vi "sosfilter.vi"() -> ()   [LabVIEW 2015]
uses:
  <vilib>/Platform/TimedLoop/XDataNode/timing_clust.ctl
  <vilib>/Platform/TimedLoop/XDataNode/nitl_modes.ctl
  <vilib>/Platform/TimedLoop/XDataNode/wakeup.ctl
  <vilib>/rvi/Emulation/niFpgaGetClockAttributes.vi
  <vilib>/rvi/Emulation/niFpgaSctlEmulationGetInTimedLoop.vi
  <vilib>/rvi/Emulation/niFpgaEmulationReportErrorSimple.vi
  <vilib>/rvi/eio/common/nirviEmuTemplateMethod_errors.vi
  <vilib>/rvi/Emulation/niFpgaEmulationIsFPGAContextNoSignature.vi
  <vilib>/rvi/errors/niFpgaSetErrorForExecOnDevCompSimple.vi
  <vilib>/rvi/eio/common/nirviEmuReportErrorAndStop.vi
  <vilib>/rvi/DataTransferAndStorage/Container/Common/niFpgaContainerGetUniqueNameForEmu.vi
  <vilib>/rvi/FIFO/Fifo_Resource/nirvififoEmulationSetSize.vi
  <vilib>/rvi/FIFO/Fifo_Resource/nirviFifoEmulationQueueMgr.vi
  <instcachedir>/0/nirviFifoEmulationQueueMgr_E5CAEC123FF24DC58D834DCA3CDAA9B5.lvgen/nirviFifoEmulationQueueMgr_E5CAEC123FF24DC58D834DCA3CDAA9B5_017.vi
  <vilib>/rvi/FIFO/Fifo_Resource/nirvififoEmulationDetermineInputValidOut.vi
  <vilib>/rvi/FIFO/Fifo_Resource/nirvififoEmulationCreateLock.vi
  <vilib>/rvi/Emulation/niFpgaProcessEmulError.vi
  <vilib>/rvi/FIFO/Fifo_Resource/nirvififoEmulationObtainLock.vi
  <vilib>/rvi/FIFO/Fifo_Resource/nirvififoEmulationReleaseLock.vi
  <vilib>/rvi/occurrence/nirviWaitOnOccurrenceBase.vi
  <vilib>/rvi/errors/nirviReportUnexpectedCaseInternalError.vi
  <vilib>/rvi/errors/nirviReportUnexpectedCaseInternalError (U32).vi
  <vilib>/rvi/Emulation/niFpgaCriticalErrorInLSC.vi
  <instcachedir>/0/nirviFifoEmulationQueueMgr_E5CAEC123FF24DC58D834DCA3CDAA9B5.lvgen/nirviFifoEmulationQueueMgr_E5CAEC123FF24DC58D834DCA3CDAA9B5_008.vi
  <vilib>/Utility/error.llb/Clear Errors.vi
  <vilib>/eio/EIONode/EIONode.xnode
  <vilib>/rvi/DataTransferAndStorage/Container/XNode/niFpgaContainer.xnode
  <vilib>/rvi/FIFO/Fifo_Resource/nirvififoEmulationWrite.vi
  <vilib>/rvi/FIFO/Fifo_Resource/nirvififoEmulationRead.vi
  <vilib>/Platform/TimedLoop/XDataNode/XDataNode.xnode
  <vilib>/rvi/FXPMathLib/FxpMul/XNode/nifxpmath_Multiplier.xnode
  <vilib>/rvi/FXPMathLib/FxpAdd/XNode/nifxpmath_Add.xnode
  <vilib>/Platform/TimedLoop/XDataNode/XDNodeRunTimeDep.lvlib
  <vilib>/rvi/FXPMathLib/sim/FxpSim.dll
panel:
  in  "a2":fxp<+/-,24,5>
  in  "b2":fxp<+/-,24,5>
  in  "b1":fxp<+/-,24,5>
  in  "a1":fxp<+/-,24,5>
  in  "b0":fxp<+/-,24,5>
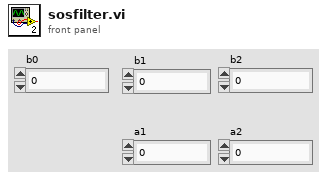
[diagram p1: front panel]
types:
  T1 = typedef "XDNodeRunTimeDep.lvlib/timing_clust.ctl" = cluster{"Expected End [f-1]":u64, "Actual End [f-1]":u64, "Finished Late? [f-1]":bool, "Expected End [i-1]":u64, "Actual End [i-1]":u64, "Finished Late? [i-1]":bool, "Expected Start [i]":u64, "Actual Start [i]":u64, "Expected Start [f]":u64, "Actual Start [f]":u64, "Source Name":string, "Structure Name":string, "Period":i64, "Deadline":i64, "Offset":i64, "Start":i64, "Priority":i32, "Timeout":i32, "Mode":T2, "Wakeup Reason":T3, "Error":errorcluster, "Source Type":string, "Secondary Source Type":string, "Global End Time":u64, "Global Start Time":u64, "Frame Duration":u64, "Iteration Duration":u64, "Assigned CPU":i32, "I/O Scan Engine Mode":u32}
  T2 = typedef "XDNodeRunTimeDep.lvlib/nitl_modes.ctl" = enum32{"No Change", "Process missed periods, maintain original phase", "Discard missed periods, maintain original phase", "Process missed periods, ignore original phase", "Discard missed periods, ignore original phase"}
  T3 = typedef "XDNodeRunTimeDep.lvlib/wakeup.ctl" = enum32{"Normal", "Aborted", "Asynchronous wakeup", "Timing source error", "Timed loop error", "Timeout"}
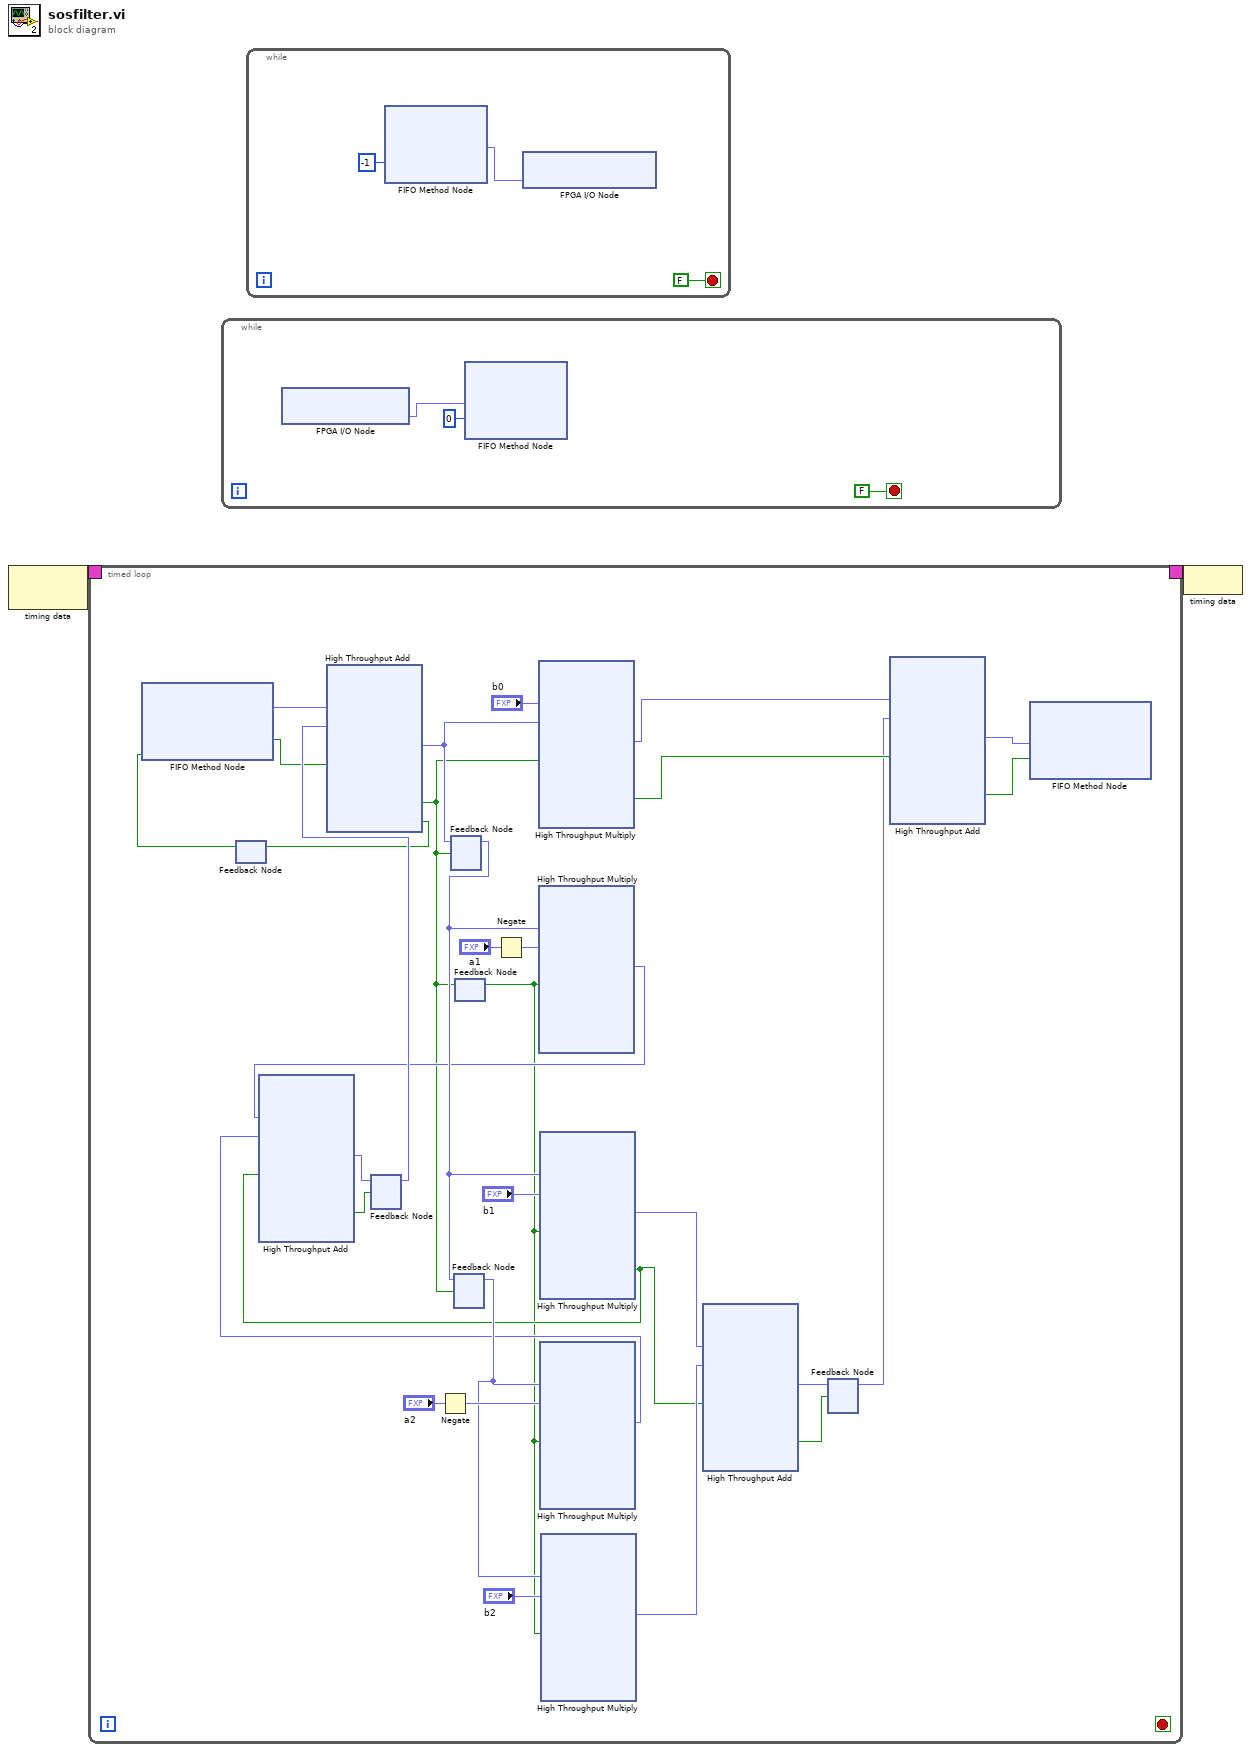
[diagram p0: block diagram]
diagram:
  n1 = node-c288() -> (w2:T1)  [unwired: 1 in]
  n2 = timed-loop {
    timing: w2 -> [_]
    timing-out: [_] -> w1
    stop <- _ stop-if-true
    n3 = feedback #1() -> (w7:bool)  [unwired: 1 in]
    n4 = xnode ("FIFO Method Node")("Ready for Output"=w7) -> ("Element"=w24:fxp<+/-,18,5>, "Output Valid"=w9:bool)  [unwired: 1 in, 1 out]
    n5 = feedback #2() -> (w19:fxp<+/-,36,16>)  [unwired: 1 in]
    n6 = xnode ("High Throughput Add")("x"=w24, "y"=w19, "input valid"=w9) -> ("x+y"=w23:fxp<+/-,36,16>, "output valid"=w13:bool, "ready for input"=w8:bool)  [unwired: 1 in]
    n7 = feedback-in #1(w8) -> ()
    n8 = Negate(x="a2") -> (-x=w27:fxp<+/-,25,6>)
    n9 = feedback-in #3(w23, w13) -> ()
    n10 = feedback #3() -> (w32:fxp<+/-,36,16>)  [unwired: 1 in]
    n11 = feedback #4() -> (w25:fxp<+/-,36,16>)  [unwired: 1 in]
    n12 = feedback-in #4(w32, w13) -> ()
    n13 = feedback-in #5(w13) -> ()
    n14 = feedback #5() -> (w12:bool)  [unwired: 1 in]
    n15 = Negate(x="a1") -> (-x=w30:fxp<+/-,25,6>)
    n16 = xnode ("High Throughput Multiply")("x"="b0", "y"=w23, "input valid"=w13) -> ("x*y"=w6:fxp<+/-,36,16>, "output valid"=w5:bool)  [unwired: 1 in, 1 out]
    n17 = xnode ("High Throughput Multiply")("x"=w32, "y"=w30, "input valid"=w12) -> ("x*y"=w18:fxp<+/-,36,16>)  [unwired: 1 in, 2 out]
    n18 = xnode ("High Throughput Multiply")("x"=w32, "y"="b1", "input valid"=w12) -> ("x*y"=w17:fxp<+/-,36,16>, "output valid"=w15:bool)  [unwired: 1 in, 1 out]
    n19 = xnode ("High Throughput Multiply")("x"=w25, "y"=w27, "input valid"=w12) -> ("x*y"=w22:fxp<+/-,36,16>)  [unwired: 1 in, 2 out]
    n20 = xnode ("High Throughput Add")("x"=w18, "y"=w22, "input valid"=w15) -> ("x+y"=w21:fxp<+/-,36,16>, "output valid"=w20:bool)  [unwired: 1 in, 1 out]
    n21 = feedback-in #2(w21, w20) -> ()
    n22 = xnode ("High Throughput Multiply")("x"=w25, "y"="b2", "input valid"=w12) -> ("x*y"=w16:fxp<+/-,36,16>)  [unwired: 1 in, 2 out]
    n23 = xnode ("High Throughput Add")("x"=w17, "y"=w16, "input valid"=w15) -> ("x+y"=w14:fxp<+/-,36,16>, "output valid"=w3:bool)  [unwired: 1 in, 1 out]
    n24 = feedback-in #6(w14, w3) -> ()
    n25 = feedback #6() -> (w4:fxp<+/-,36,16>)  [unwired: 1 in]
    n26 = xnode ("High Throughput Add")("x"=w6, "y"=w4, "input valid"=w5) -> ("x+y"=w11:fxp<+/-,36,16>, "output valid"=w10:bool)  [unwired: 1 in, 1 out]
    n27 = xnode ("FIFO Method Node")("Element"=w11, "Input Valid"=w10) -> ()  [unwired: 1 in, 2 out]
  }
  n28 = while {
    stop <- FALSE stop-if-true
    n29 = xnode "FPGA I/O Node"() -> ("Connector0/AI0"=w38:fxp<+/-,27,5>)  [unwired: 1 in, 1 out]
    n30 = xnode ("FIFO Method Node")("Element"=w38, "Timeout"=0) -> ()  [unwired: 1 in, 2 out]
  }
  n31 = while {
    stop <- FALSE stop-if-true
    n32 = xnode ("FIFO Method Node")("Timeout"=-1) -> ("Element"=w39:fxp<+/-,20,5>)  [unwired: 1 in, 2 out]
    n33 = xnode "FPGA I/O Node"("Connector0/AO0"=w39) -> ()  [unwired: 1 in, 1 out]
  }
  n34 = node-c288(w1) -> ()
